vi "Slop Adjustment.vi"(9 "Slop Measure":dbl=5.0, 10 "Adjustment":dbl, 11 "Setpoint":dbl) -> (3 "Adjusted Setpoint":dbl)   [LabVIEW 2019]
uses:
  GlobalVariables.vi
panel:
  out "Previous State":bool
  out "Slop Location":bool
  # "Practice Bot is 5 Degrees of Slop"
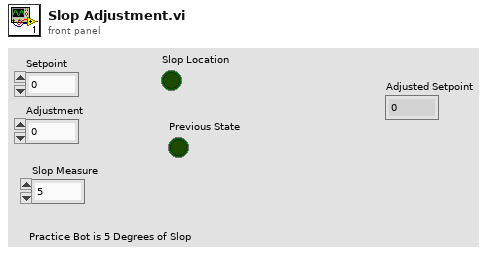
[diagram p1: front panel]
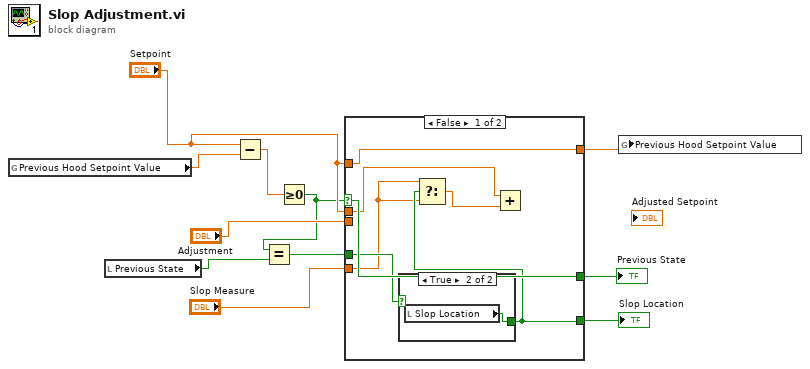
[diagram p0: block diagram]
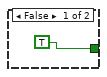
[diagram p2: hidden frame]
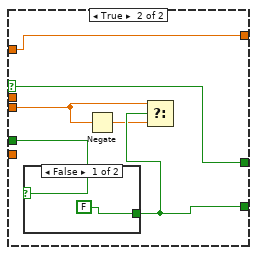
[diagram p3: hidden frame]
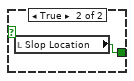
[diagram p4: hidden frame]
diagram:
  n1 = global read "GlobalVariables.vi" "Previous Hood Setpoint Value"() -> (w11:dbl)
  n2 = local read "Previous State"() -> (w2:bool)
  n3 = Subtract(x="Setpoint", y=w11) -> (x-y=w10:dbl)
  n4 = Greater Or Equal To 0?(x=w10) -> (x >= 0?=w5:bool)
  n5 = Equal?(x=w5, y=w2) -> (x = y?=w4:bool)
  n6 = case shown="False" w5 {
    selector: w5 -> [w17 w25]
    tunnel: "Setpoint" -> [w18 w26]
    tunnel: [w18 w26] -> w9
    tunnel: "Setpoint" -> [w12 _]
    tunnel: "Adjustment" -> [_ w22]
    tunnel: [w17 w25] -> w6
    tunnel: w4 -> [w16 w24]
    tunnel: [w15 w23] -> w3
    tunnel: "Slop Measure" -> [w14 _]
    frame False {
      n7 = case shown="True" w16 {
        tunnel: [TRUE w20] -> w15
        frame False {
        }
        frame True {
          n8 = local read "Slop Location"() -> (w20:bool)
        }
      }
      n9 = Select(t=w14, s=w15, f=w14) -> (s? t:f=w13:dbl)
      n10 = Add(x=w12, y=w13) -> ()  [unwired: 1 out]
    }
    frame True {
      n11 = case shown="False" w24 {
        tunnel: [FALSE w28] -> w23
        frame False {
        }
        frame True {
          n12 = local read "Slop Location"() -> (w28:bool)
        }
      }
      n13 = Negate(x=w22) -> (-x=w21:dbl)
      n14 = Select(t=w22, s=w23, f=w21) -> ()  [unwired: 1 out]
    }
  }
  "Slop Location" <- w3
  "Previous State" <- w6
  n15 = global write "GlobalVariables.vi" "Previous Hood Setpoint Value"(w9) -> ()
